vi "Log Sweep.vi"(8 "error in (no error)":errorcluster, 10 "SweepWaveforms":T1, 11 "Instrument.Lockin in":refnum<class "Instrument.Lockin.lvclass">) -> (0 "error out":errorcluster)   [LabVIEW 2019, in "Instrument.Lockin.lvlib" / "Instrument.Lockin.lvclass"]
uses:
  Instrument.Lockin.lvclass
  C:/Program Files/National Instruments/LabVIEW 2019/user.lib/LevyLab/Instrument Framework/Instrument/Instrument.lvclass
  Instrument.DAQ/Typedefs/PublicEvents--DAQ.getSweepWaveforms.ctl
  <userlib>/LevyLab/Instrument Framework/Instrument/Instrument.lvclass
  Instrument.DAQ/Instrument.DAQ.lvclass
panel:
  out "Instrument.Lockin out":refnum<class "Instrument.Lockin.lvclass">
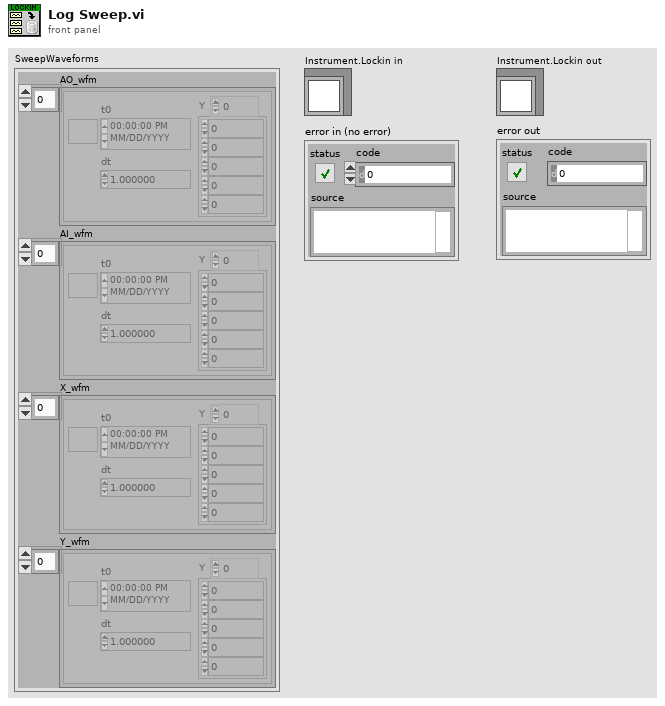
[diagram p1: front panel]
types:
  T1 = typedef "Instrument.Lockin.lvlib/Instrument.DAQ.lvclass/PublicEvents--DAQ.getSweepWaveforms.ctl" = cluster{"AO_wfm":waveform(dbl)[], "AI_wfm":waveform(dbl)[], "X_wfm":waveform(dbl)[], "Y_wfm":waveform(dbl)[]}
  T2 = typedef "Instrument.Lockin.lvlib/Instrument.Lockin.lvclass/Lockin.LogSweepAOAI--Cluster.ctl" = cluster{"ChassisSerialNumber":u32, "Channel":i32, "Data":dbl, "Sweeping?":bool}
  T3 = typedef "Instrument.Lockin.lvlib/Instrument.Lockin.lvclass/Lockin.LogSweepXY--Cluster.ctl" = cluster{"ChassisSerialNumber":u32, "Channel":i32, "REF Channel":i32, "X":dbl, "Y":dbl, "Sweeping?":bool}
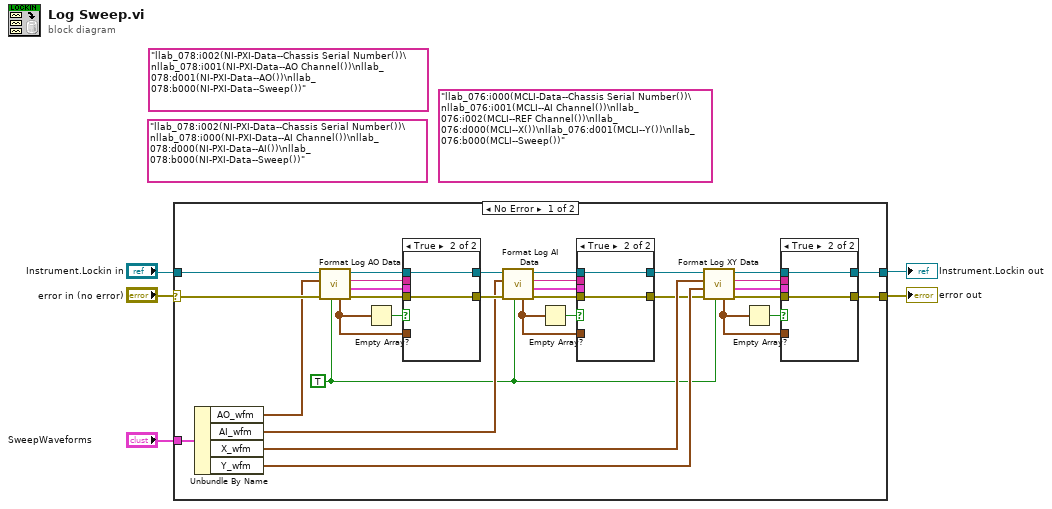
[diagram p0: block diagram]
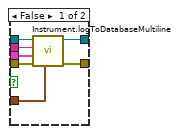
[diagram p2: hidden frame]
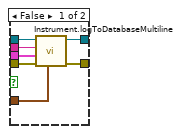
[diagram p3: hidden frame]
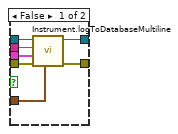
[diagram p4: hidden frame]
diagram:
  (unwired) "llab_078:i002(NI-PXI-Data--Chassis Serial Number())\nllab_078:i001(NI-PXI-Data--AO Channel())\nllab_078:d001(NI-PXI-Data--AO())\nllab_078:b000(NI-PXI-Data--Sweep())"
  (unwired) "llab_078:i002(NI-PXI-Data--Chassis Serial Number())\nllab_078:i000(NI-PXI-Data--AI Channel())\nllab_078:d000(NI-PXI-Data--AI())\nllab_078:b000(NI-PXI-Data--Sweep())"
  (unwired) "llab_076:i000(MCLI-Data--Chassis Serial Number())\nllab_076:i001(MCLI--AI Channel())\nllab_076:i002(MCLI--REF Channel())\nllab_076:d000(MCLI--X())\nllab_076:d001(MCLI--Y())\nllab_076:b000(MCLI--Sweep())"
  n1 = case shown="No Error" "error in (no error)" {
    selector: "error in (no error)" -> [w35 w66]
    tunnel: "Instrument.Lockin in" -> [w37 w65]
    tunnel: [w34 w66] -> w5
    tunnel: "SweepWaveforms" -> [w36 _]
    tunnel: [w33 w65] -> w2
    frame No Error {
      w12 = TRUE ("Sweeping?")
      n2 = Unbundle By Name(w36) -> ("AO_wfm"=w32:waveform(dbl)[], "AI_wfm"=w25:waveform(dbl)[], "X_wfm"=w15:waveform(dbl)[], "Y_wfm"=w14:waveform(dbl)[])
      n3 = call "Format Log AO Data.vi"("Sweeping?"=w12, "error in (no error)"=w35, "waveform"=w32, "Instrument.Lockin in"=w37) -> ("error out"=w29:errorcluster, "Log Data"=w22:T2[], "Log Paths"=w21:string, "Instrument.Lockin out"=w31:refnum<class "Instrument.Lockin.lvclass">, "Times"=w30:timestamp[])  [unwired: 3 in]
      n4 = Empty Array?(array=w30) -> (empty?=w28:bool)
      n5 = case shown="True" w28 {
        tunnel: w31 -> [w62 w64]
        tunnel: w30 -> [w61 _]
        tunnel: w29 -> [w60 w63]
        tunnel: [w59 w64] -> w27
        tunnel: [w58 w63] -> w26
        tunnel: w22 -> [w57 _]
        tunnel: w21 -> [w56 _]
        frame False {
          n6 = call <userlib>:"Instrument.logToDatabaseMultiline.vi"("timestamps"=w61, "error in (no error)"=w60, "Data"=w57, "Paths"=w56, "Instrument"=w62) -> ("error out"=w58:errorcluster, "Instrument out"=w59:refnum<class "Instrument.Lockin.lvclass">)  [unwired: 5 in]
        }
        frame True {
        }
      }
      n7 = call "Format Log AI Data.vi"("Sweeping?"=w12, "error in (no error)"=w26, "waveform"=w25, "Instrument.Lockin in"=w27) -> ("error out"=w18:errorcluster, "Log Data"=w20:T2[], "Log Paths"=w19:string, "Instrument.Lockin out"=w23:refnum<class "Instrument.Lockin.lvclass">, "Times"=w17:timestamp[])  [unwired: 3 in]
      n8 = Empty Array?(array=w17) -> (empty?=w24:bool)
      n9 = case shown="True" w24 {
        tunnel: w23 -> [w53 w55]
        tunnel: w17 -> [w52 _]
        tunnel: w18 -> [w51 w54]
        tunnel: [w50 w55] -> w16
        tunnel: [w49 w54] -> w13
        tunnel: w20 -> [w48 _]
        tunnel: w19 -> [w47 _]
        frame False {
          n10 = call <userlib>:"Instrument.logToDatabaseMultiline.vi"("timestamps"=w52, "error in (no error)"=w51, "Data"=w48, "Paths"=w47, "Instrument"=w53) -> ("error out"=w49:errorcluster, "Instrument out"=w50:refnum<class "Instrument.Lockin.lvclass">)  [unwired: 5 in]
        }
        frame True {
        }
      }
      n11 = call "Format Log XY Data.vi"("Sweeping?"=w12, "error in (no error)"=w13, "Y"=w14, "X"=w15, "Instrument.Lockin in"=w16) -> ("error out"=w7:errorcluster, "Log Data"=w9:T3[], "Log Paths"=w8:string, "Instrument.Lockin out"=w10:refnum<class "Instrument.Lockin.lvclass">, "Times"=w6:timestamp[])  [unwired: 2 in]
      n12 = Empty Array?(array=w6) -> (empty?=w11:bool)
      n13 = case shown="True" w11 {
        tunnel: w10 -> [w44 w46]
        tunnel: w6 -> [w43 _]
        tunnel: w7 -> [w42 w45]
        tunnel: [w41 w46] -> w33
        tunnel: [w40 w45] -> w34
        tunnel: w9 -> [w39 _]
        tunnel: w8 -> [w38 _]
        frame False {
          n14 = call <userlib>:"Instrument.logToDatabaseMultiline.vi"("timestamps"=w43, "error in (no error)"=w42, "Data"=w39, "Paths"=w38, "Instrument"=w44) -> ("error out"=w40:errorcluster, "Instrument out"=w41:refnum<class "Instrument.Lockin.lvclass">)  [unwired: 5 in]
        }
        frame True {
        }
      }
    }
    frame Error {
    }
  }
  "error out" <- w5
  "Instrument.Lockin out" <- w2
